vi "Configuration.WavelengthSweeping.Writer.Test.vi"() -> ()   [LabVIEW 2017, in "Measurement.WavelengthSweeping.lvclass"]
uses:
  Measurement.WavelengthSweeping.lvclass
  Typedefs/Configuration--Cluster.ctl
  Measurement/Typedefs/Measurement.Type--Enum.ctl
  Typedefs/Configuration.Hardware--Cluster.ctl
  Measurement/Typedefs/Configuration.SMU--Cluster.ctl
  SMU/Typedefs/Configuration--Cluster.ctl
  Measurement/Typedefs/Configuration.LIA--Cluster.ctl
  LIA/Typedefs/Configuration--Cluster.ctl
  Measurement/Typedefs/Configuration.OPM--Cluster.ctl
  OPM/Typedefs/Configuration--Cluster.ctl
  Measurement/Typedefs/Configuration.OPA--Cluster.ctl
  OPA/Typedefs/Configuration--Cluster.ctl
  Typedefs/Configuration.Measurement--Cluster.ctl
  <vilib>/Utility/config.llb/NI_LVConfig.lvlib
  Measurement/Measurement.lvclass
  SMU/SMU.lvclass
  LIA/LIA.lvclass
  OPM/OPM.lvclass
  OPA/OPA.lvclass
panel:
  out "error out":errorcluster
  in  "Configuration.WavelengthSweeping":T1={"Measurement.Type"=enum."Wavelength sweeping", "Configuration.Hardware"={"SMU"={"Enable"=TRUE, "SMU Model"="Keithley2600", "Configuration"={"VISA Resource"="GPIB0::26::INSTR", "Channel"="A"}}, "LIA"={"Enable"=TRUE, "LIA Model"="SR810", "Configuration"={"VISA Resource"="GPIB0::8::INSTR"}}, "OPM"={"Enable"=TRUE, "OPM Model"="ThorlabsPM400", "Configuration"={"VISA Resource"="USB0::0x1313::0x8075::P5001221::INSTR"}}, "OPA"={"Enable"=TRUE, "OPA Model"="OrpheusHP", "Configuration"={"Serial Number"="Orpheus-HP-Demo-8047"}}}, "Configuration.Measurement"={"SMU Voltage, V"=1.0, "OPA Start wavelength, nm"=600.0, "OPA Stop wavelength, nm"=1000.0, "OPA Scan resolution, nm"=20.0, "OPA Number or points"=0, "Integration time, sec"=1.0, "Delay time, ms"=100, "Accumulation"=5}}
  # "e"
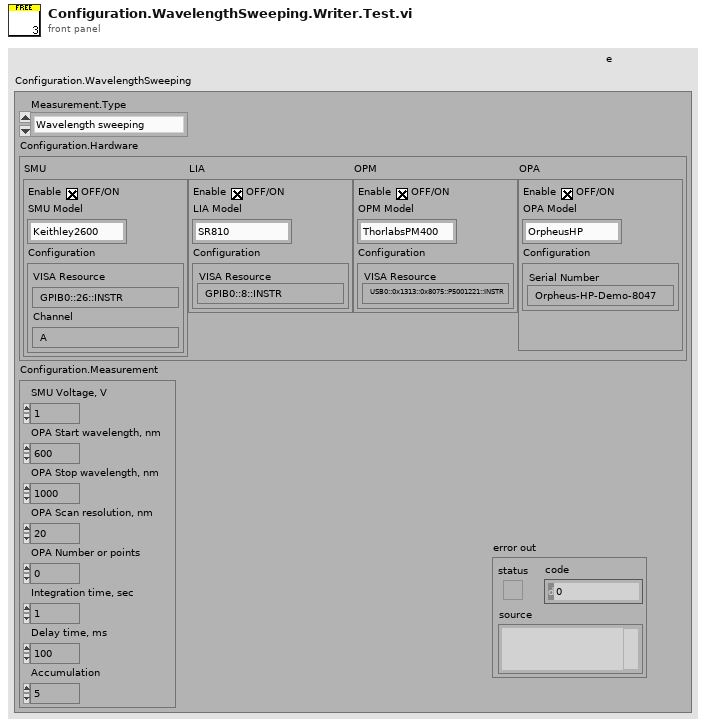
[diagram p1: front panel]
types:
  T1 = typedef "Measurement.WavelengthSweeping.lvclass/Configuration--Cluster.ctl" = cluster{"Measurement.Type":T2, "Configuration.Hardware":T3, "Configuration.Measurement":T12}
  T2 = typedef "Measurement.lvclass/Measurement.Type--Enum.ctl" = enum16{"Free", "I/V Curve", "Wavelength sweeping", "Photocurrent mapping"}
  T3 = typedef "Measurement.WavelengthSweeping.lvclass/Configuration.Hardware--Cluster.ctl" = cluster{"SMU":T4, "LIA":T6, "OPM":T8, "OPA":T10}
  T4 = typedef "Measurement.lvclass/Configuration.SMU--Cluster.ctl" = cluster{"Enable":bool, "SMU Model":string, "Configuration":T5}
  T5 = typedef "SMU.lvclass/Configuration--Cluster.ctl" = cluster{"VISA Resource":string, "Channel":string}
  T6 = typedef "Measurement.lvclass/Configuration.LIA--Cluster.ctl" = cluster{"Enable":bool, "LIA Model":string, "Configuration":T7}
  T7 = typedef "LIA.lvclass/Configuration--Cluster.ctl" = cluster{"VISA Resource":string}
  T8 = typedef "Measurement.lvclass/Configuration.OPM--Cluster.ctl" = cluster{"Enable":bool, "OPM Model":string, "Configuration":T9}
  T9 = typedef "OPM.lvclass/Configuration--Cluster.ctl" = cluster{"VISA Resource":string}
  T10 = typedef "Measurement.lvclass/Configuration.OPA--Cluster.ctl" = cluster{"Enable":bool, "OPA Model":string, "Configuration":T11}
  T11 = typedef "OPA.lvclass/Configuration--Cluster.ctl" = cluster{"Serial Number":string}
  T12 = typedef "Measurement.WavelengthSweeping.lvclass/Configuration.Measurement--Cluster.ctl" = cluster{"SMU Voltage, V":dbl, "OPA Start wavelength, nm":dbl, "OPA Stop wavelength, nm":dbl, "OPA Scan resolution, nm":dbl, "OPA Number or points":u16, "Integration time, sec":dbl, "Delay time, ms":u16, "Accumulation":u16}
  T13 = typedef "NI_LVConfig.lvlib/Config Data RefNum.ctl" = refnum<k1>
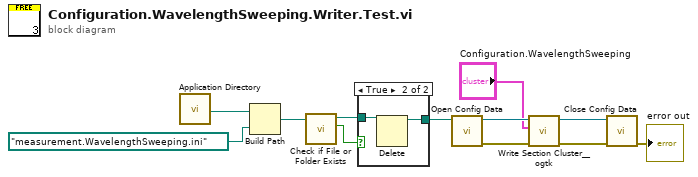
[diagram p0: block diagram]
diagram:
  n1 = call <vilib>:"Application Directory.vi"() -> ("Application Directory"=w12:path)
  n2 = Build Path(base path=w12, name or relative path=path "measurement.WavelengthSweeping.ini") -> (appended path=w3:path)
  n3 = call <vilib>:"Check if File or Folder Exists.vi"("path"=w3) -> ("file or folder exists?"=w1:bool, "dup path"=w2:path)  [unwired: 8 in, 1 out]
  n4 = case shown="True" w1 {
    tunnel: [w13 w15] -> w5
    tunnel: w2 -> [w13 w14]
    frame False {
    }
    frame True {
      n5 = Delete(path (use dialog)=w14) -> (deleted path=w15:path)  [unwired: 4 in, 2 out]
    }
  }
  n6 = call <vilib>:"Open Config Data.vi"("configuration file path"=w5) -> ("error out"=w10:errorcluster, "refnum"=w7:T13)  [unwired: 8 in, 1 out]
  n7 = call <userlib>:"Write Section Cluster__ogtk.vi"("error in (no error)"=w10, "Section Formatted Cluster"="Configuration.WavelengthSweeping", "refnum"=w7) -> ("error out"=w9:errorcluster, "dup refnum"=w8:T13)  [unwired: 7 in]
  n8 = call <vilib>:"Close Config Data.vi"("error in (no error)"=w9, "refnum"=w8) -> ("error out"=→"error out":errorcluster)  [unwired: 8 in, 1 out]
